vi "_CreateReply.vi"(3 "Ring":T1 items=["FullUpdate", "RefeeChanged", "AdaptToInputs", "Refresh", "FontChange"]) -> (1 "Reply":string[](array[string]))   [LabVIEW 2020, in "XDataNode.xnode"]
uses:
  XDataNode.xnode
  ReplySet.ctl
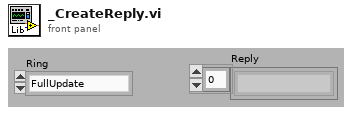
[diagram p1: front panel]
types:
  T1 = typedef "XDataNode.xnode/ReplySet.ctl" = u16
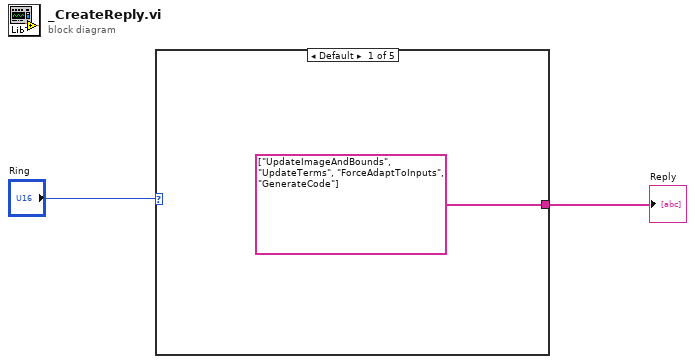
[diagram p0: block diagram]
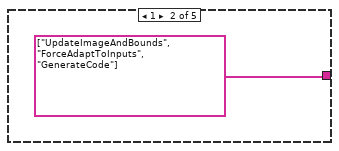
[diagram p2: hidden frame]
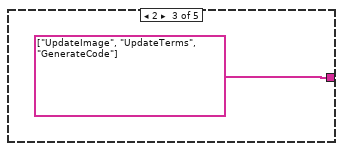
[diagram p3: hidden frame]
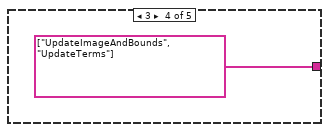
[diagram p4: hidden frame]
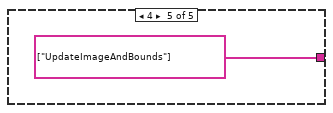
[diagram p5: hidden frame]
diagram:
  n1 = case shown="Default" "Ring" {
    tunnel: [string[] ["UpdateImageAndBounds", "UpdateTerms", "ForceAdaptToInputs", "GenerateCode"] ("Reply") string[] ["UpdateImageAndBounds", "ForceAdaptToInputs", "GenerateCode"] ("Reply") string[] ["UpdateImage", "UpdateTerms", "GenerateCode"] ("Reply") string[] ["UpdateImageAndBounds", "UpdateTerms"] ("Reply") string[] ["UpdateImageAndBounds"] ("Reply")] -> w2
    frame Default {
    }
    frame 1 {
    }
    frame 2 {
    }
    frame 3 {
    }
    frame 4 {
    }
  }
  "Reply" <- w2
